vi "Panel Split Engine.vi"() -> ()   [LabVIEW 2016]
uses:
  PanelRootNode.lvclass
  QueueManager.llb/Destroy.vi
  QueueManager.llb/Remove.vi
  PanelDataNode/PanelDataNode.lvclass
  QueueManager.llb/CreatQueue.vi
  <vilib>/Utility/error.llb/DialogType.ctl
panel:
  out "RootNode*":refnum<data-value>
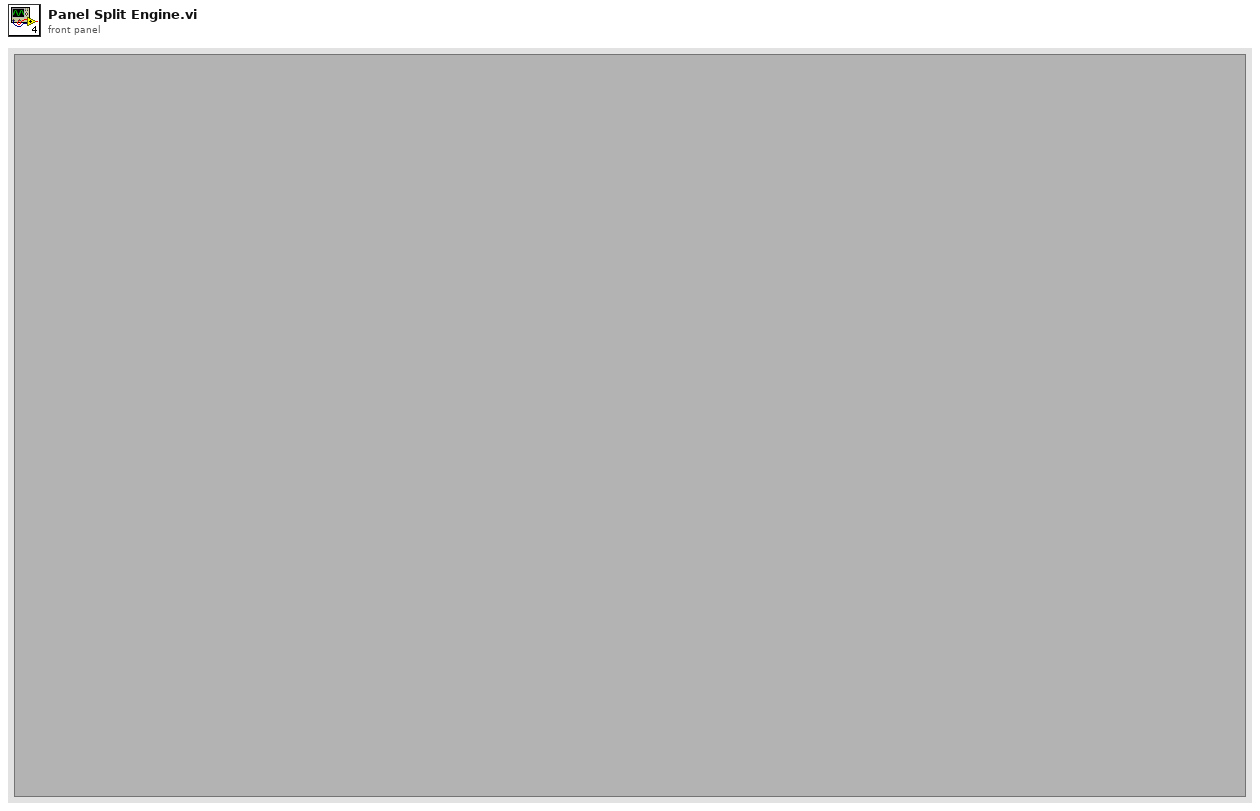
[diagram p1: front panel]
types:
  T1 = cluster{"error":errorcluster, "Event":string, "Data":variant, "Q_Local":string, "RootNode*":refnum<data-value>, "Caller":string}
  T2 = typedef "DialogType.ctl" = u16
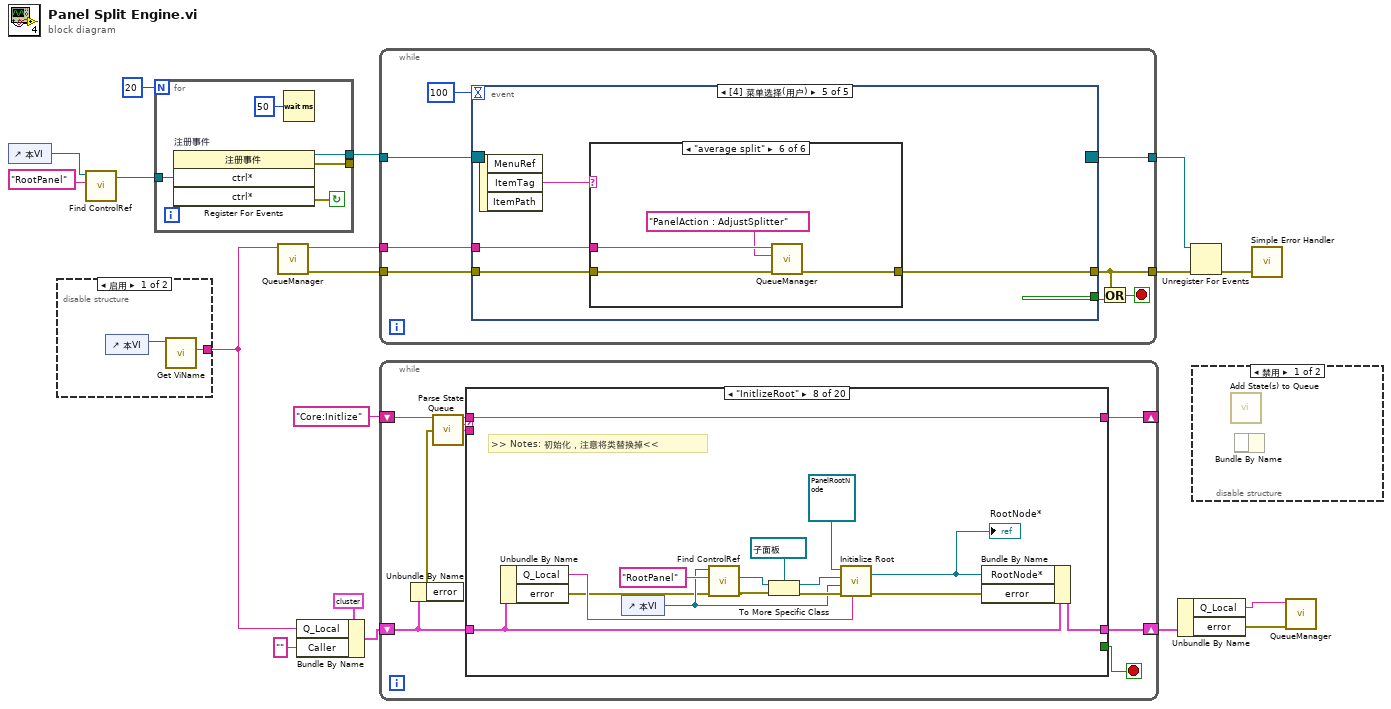
[diagram p0: block diagram]
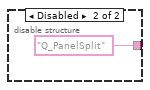
[diagram p2: hidden frame]
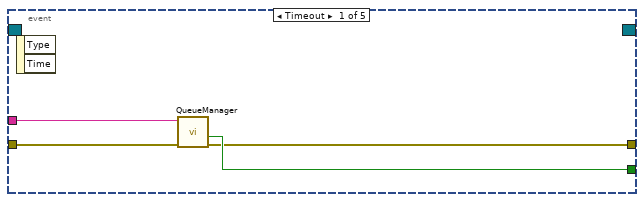
[diagram p4: hidden frame]
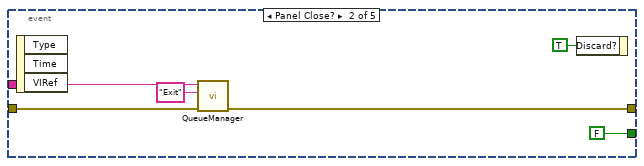
[diagram p5: hidden frame]
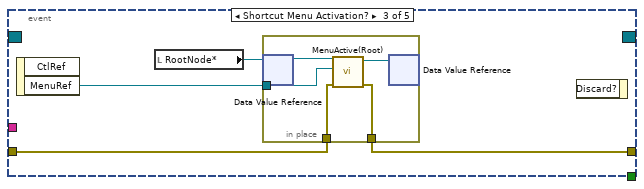
[diagram p6: hidden frame]
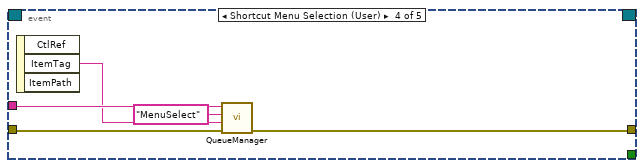
[diagram p7: hidden frame]
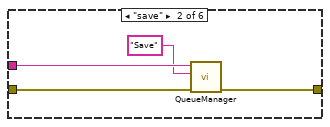
[diagram p9: hidden frame]
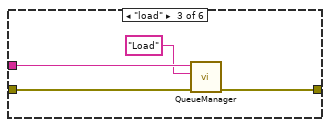
[diagram p10: hidden frame]
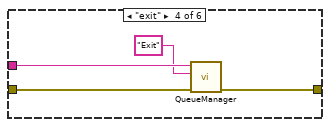
[diagram p11: hidden frame]
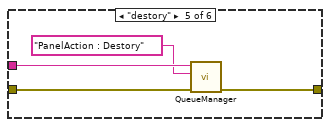
[diagram p12: hidden frame]
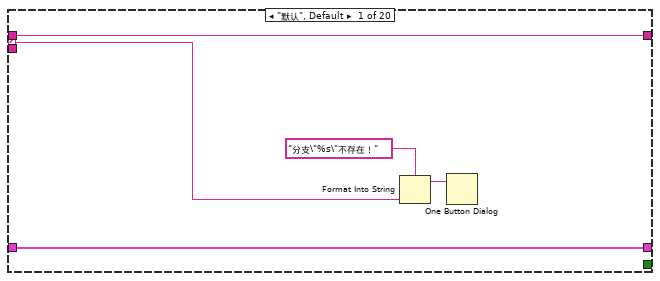
[diagram p13: hidden frame]
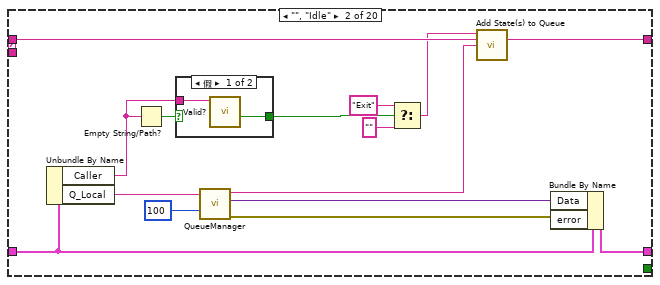
[diagram p14: hidden frame]
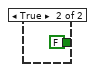
[diagram p15: hidden frame]
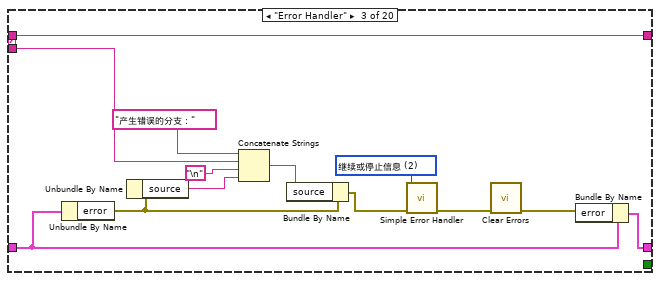
[diagram p16: hidden frame]
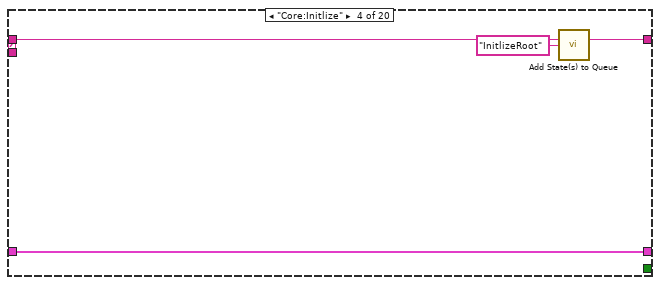
[diagram p17: hidden frame]
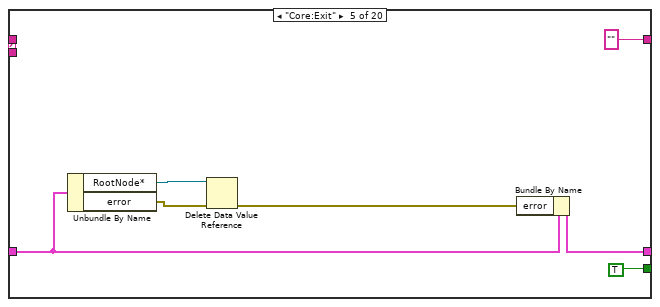
[diagram p18: hidden frame]
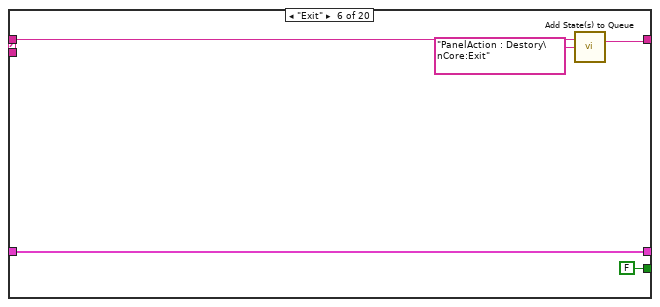
[diagram p19: hidden frame]
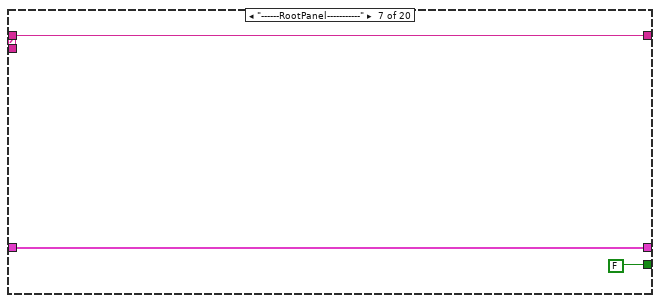
[diagram p20: hidden frame]
diagram:
  n1 = control-ref of="本VI"() -> (w8:refnum<vi>)
  n2 = disable-structure shown="启用" {
    disable-tunnel: [w18 "Q_PanelSplit" ("QueueName")] -> w10
    frame Enabled {
      n3 = control-ref of="本VI"() -> (w19:refnum<vi>)
      n4 = call "Get ViName.vi"("VI*"=w19) -> ("VI Name"=w18:string)  [unwired: 8 in, 2 out]
    }
    frame Disabled {
    }
  }
  n5 = call "Find ControlRef.vi"("control name"="RootPanel", "vi*"=w8) -> ("ctrl*"=w2:refnum<vi>)  [unwired: 7 in, 2 out]
  n6 = for {
    N: 20 -> [_]
    tunnel: [w22] -> _
    tunnel: [w24] -> w3
    tunnel: w2 -> [w23]
    stop <- w22 continue-if-true
    n7 = register-events "注册事件"(w23, w23) -> (reference out=w24:refnum<event-registration>, error out=w22:errorcluster)  [unwired: 2 in]
    n8 = Wait (ms)(milliseconds to wait=u32 50 ("等待时间（毫秒）")) -> ()  [unwired: 1 out]
  }
  n9 = call-poly "QueueManager.vi"("QueueName"=w10) -> ("error out"=w17:errorcluster)  [unwired: 9 in, 1 out]
  n10 = Bundle By Name(cluster=T1 {"error"={"status"=FALSE, "code"=0, "source"=""}, "Event"="", "Data"=variant, "Q_Local"="", "RootNode*"=refnum, "Caller"=""} ("TmpData"), "Q_Local"=w10, "Caller"="") -> (w12:T1)
  n11 = while {
    tunnel: w17 -> [w31]
    tunnel: w10 -> [w32]
    tunnel: [w28] -> w6
    tunnel: w3 -> [w26]
    tunnel: [w25] -> w4
    stop <- w29 stop-if-true
    n12 = event shown="[4] 菜单选择(用户)" {
      selector: w26 -> [_ _ _ _ _]
      dyn-events: [_ _ _ _ _] -> w25
      timeout: 100 -> [_ _ _ _ _]
      tunnel: [w34 FALSE _ _ _] -> w30
      tunnel: w32 -> [w36 w41 _ w56 w59]
      tunnel: w31 -> [w35 w40 w45 w55 w58]
      tunnel: [w33 w39 w46 w54 w57] -> w28
      event Timeout {
        n13 = event-data() -> ()  [unwired: 1 in, 2 out]
        n14 = call-poly "QueueManager.vi"("error in (no error)"=w35, "Queue Name(unamed)"=w36) -> ("error out"=w33:errorcluster, "Not Exist?"=w34:bool)  [unwired: 8 in]
      }
      event Panel Close? {
        n15 = event-data() -> ()  [unwired: 1 in, 3 out]
        n16 = call-poly "QueueManager.vi"("error in"=w40, "Event"="Exit", "QueueName"=w41) -> ("error out"=w39:errorcluster)  [unwired: 7 in, 1 out]
        n17 = event-data("Discard?"=TRUE ("放弃？")) -> ()  [unwired: 1 in, 1 out]
      }
      event Shortcut Menu Activation? {
        n18 = event-data() -> ("MenuRef"=w44:refnum<k9>)  [unwired: 1 in, 1 out]
        n19 = local read "RootNode*"() -> (w43:refnum<data-value>)
        n20 = in-place {
          in-place-border: w44 -> [w49]
          in-place-border: w45 -> [w48]
          in-place-border: [w47] -> w46
          n21 = in-place-dvr #1(w43) -> (w51:refnum<class "PanelRootNode.lvclass">)  [unwired: 1 out]
          n22 = call "MenuActive(Root).vi"("error in (no error)"=w48, "菜单引用"=w49, "PanelDataNode 输入"=w51) -> ("error out"=w47:errorcluster, "PanelDataNode 输出"=w50:refnum<class "PanelRootNode.lvclass">)  [unwired: 7 in]
          n23 = in-place-dvr #1(w50) -> ()  [unwired: 2 out]
        }
        n24 = event-data() -> ()  [unwired: 2 in, 1 out]
      }
      event Shortcut Menu Selection (User) {
        n25 = event-data() -> ("ItemTag"=w53:string)  [unwired: 1 in, 2 out]
        n26 = call-poly "QueueManager.vi"("error in"=w55, "Data"=w53, "Event"="MenuSelect", "QueueName"=w56) -> ("error out"=w54:errorcluster)  [unwired: 6 in, 1 out]
      }
      event Menu Selection (User) {
        n27 = event-data() -> ("ItemTag"=w60:string)  [unwired: 1 in, 2 out]
        n28 = case shown="\"average split\"" w60 {
          tunnel: w59 -> [_ w65 w69 w73 w77 w81]
          tunnel: w58 -> [w61 w63 w67 w71 w75 w79]
          tunnel: [w61 w62 w66 w70 w74 w78] -> w57
          frame "假", Default {
          }
          frame "save" {
            n29 = call-poly "QueueManager.vi"("error in"=w63, "Event"="Save", "QueueName"=w65) -> ("error out"=w62:errorcluster)  [unwired: 7 in, 1 out]
          }
          frame "load" {
            n30 = call-poly "QueueManager.vi"("error in"=w67, "Event"="Load", "QueueName"=w69) -> ("error out"=w66:errorcluster)  [unwired: 7 in, 1 out]
          }
          frame "exit" {
            n31 = call-poly "QueueManager.vi"("error in"=w71, "Event"="Exit", "QueueName"=w73) -> ("error out"=w70:errorcluster)  [unwired: 7 in, 1 out]
          }
          frame "destory" {
            n32 = call-poly "QueueManager.vi"("error in"=w75, "Event"="PanelAction : Destory", "QueueName"=w77) -> ("error out"=w74:errorcluster)  [unwired: 7 in, 1 out]
          }
          frame "average split" {
            n33 = call-poly "QueueManager.vi"("error in"=w79, "Event"="PanelAction : AdjustSplitter", "QueueName"=w81) -> ("error out"=w78:errorcluster)  [unwired: 7 in, 1 out]
          }
        }
      }
    }
    n34 = Or(x=w28, y=w30) -> (x .or. y?=w29:bool)
  }
  n35 = while {
    shift-right: [w83] -> w14
    shift-left: w12 -> [w84]
    shift-right: [w82] -> _
    shift-left: "Core:Initlize" -> [w90]
    stop <- w86 stop-if-true
    n36 = Unbundle By Name(w84) -> ("error"=w85:errorcluster)
    n37 = call "Parse State Queue.vi"("State Queue"=w90, "Error In (no error)"=w85) -> ("Remaining States"=w89:string, "Current State"=w88:string, "Arguments"=w87:string)  [unwired: 10 in, 1 out]
    n38 = case shown="\"InitlizeRoot\"" w88 {
      selector: w88 -> [w91 _ _ _ _ _ _ _ _ _ _ _ _ _ _ _ _ _ _ _]
      tunnel: w89 -> [w94 w106 w126 w129 _ w142 w143 w160 w168 w189 w207 w219 w230 w237 w248 w258 w268 w278 w284 w296]
      tunnel: w87 -> [_ _ w114 _ _ _ _ _ _ _ _ _ _ _ _ _ _ _ _ _]
      tunnel: [_ _ _ _ TRUE FALSE FALSE _ _ _ _ _ _ _ _ _ _ _ _ _] -> w86
      tunnel: w84 -> [w95 w103 w116 w130 w133 w139 w144 w152 w170 w187 w205 w223 w229 w236 w246 w256 w266 w276 w283 w294]
      tunnel: [w95 w109 w115 w130 w132 w139 w144 w154 w169 w186 w204 w222 w229 w235 w245 w255 w265 w275 w283 w293] -> w83
      tunnel: [w94 w105 w126 w128 "" ("Remaining States") w141 w143 w160 w168 w189 w207 w218 w230 w237 w248 w258 w268 w278 w284 w296] -> w82
      frame "默认", Default {
        n39 = Format Into String(format string="分支\"%s\"不存在！" ("格式字符串"), w91) -> (resulting string=w93:string)  [unwired: 2 in, 1 out]
        n40 = One Button Dialog(message=w93) -> ()  [unwired: 1 in, 1 out]
      }
      frame "", "Idle" {
        n41 = Unbundle By Name(w103) -> ("Caller"=w97:string, "Q_Local"=w102:string)
        n42 = Empty String/Path?(string/path=w97) -> (empty?=w101:bool)
        n43 = case shown="假" w101 {
          tunnel: [w112 FALSE ("Not Exist?")] -> w100
          tunnel: w97 -> [w111 _]
          frame False {
            n44 = call "Valid?.vi"("Queue Name(unamed)"=w111) -> ("Not Exist?"=w112:bool)  [unwired: 9 in, 1 out]
          }
          frame True {
          }
        }
        n45 = call-poly "QueueManager.vi"("Time out(-1)"=100, "Queue Name"=w102) -> ("error out"=w110:errorcluster, "Data"=w108:variant, "Event"=w107:string)  [unwired: 6 in, 1 out]
        n46 = Select(t="Exit" ("Event"), s=w100, f="") -> (s? t:f=w96:string)
        n47 = call "Add State(s) to Queue.vi"("State(s) in Front (\"\")"=w96, "State(s) in (\"\")"=w106, "State(s) at Back (\"\")"=w107) -> ("States Out"=w105:string)  [unwired: 12 in]
        n48 = Bundle By Name(cluster=w103, "Data"=w108, "error"=w110) -> (w109:T1)
      }
      frame "Error Handler" {
        w123 = T2 2 items=["无对话框", "确定信息", "继续或停止信息", "确定信息＋警告", "继续/停止+警告"] ("type of dialog (OK msg:1)")
        n49 = Unbundle By Name(w116) -> ("error"=w118:errorcluster)
        n50 = Unbundle By Name(w118) -> ("source"=w121:string)
        n51 = Concatenate Strings("产生错误的分支：" ("字符串"), w114, "\n", w121) -> (w119:string)
        n52 = Bundle By Name(cluster=w118, "source"=w119) -> (w117:errorcluster)
        n53 = call <vilib>:"Simple Error Handler.vi"("type of dialog (OK msg:1)"=w123, "error in (no error)"=w117) -> ("error out"=w124:errorcluster)  [unwired: 3 in, 4 out]
        n54 = call <vilib>:"Clear Errors.vi"("error in (no error)"=w124) -> ("error out"=w125:errorcluster)  [unwired: 5 in, 1 out]
        n55 = Bundle By Name(cluster=w116, "error"=w125) -> (w115:T1)
      }
      frame "Core:Initlize" {
        n56 = call "Add State(s) to Queue.vi"("State(s) in (\"\")"=w129, "State(s) at Back (\"\")"="InitlizeRoot" ("State(s) at Back (\"\")")) -> ("States Out"=w128:string)  [unwired: 13 in]
      }
      frame "Core:Exit" {
        n57 = Unbundle By Name(w133) -> ("RootNode*"=w135:refnum<data-value>, "error"=w131:errorcluster)
        n58 = Delete Data Value Reference(data value reference=w135, error in=w131) -> (error out=w134:errorcluster)  [unwired: 1 out]
        n59 = Bundle By Name(cluster=w133, "error"=w134) -> (w132:T1)
      }
      frame "Exit" {
        n60 = call "Add State(s) to Queue.vi"("State(s) in (\"\")"=w142, "State(s) at Back (\"\")"="PanelAction : Destory\nCore:Exit" ("State(s) at Back (\"\")")) -> ("States Out"=w141:string)  [unwired: 13 in]
      }
      frame "------RootPanel-----------" {
      }
      frame "InitlizeRoot" {
        # ">> Notes: 初始化，注意将类替换掉<<"
        n61 = Unbundle By Name(w152) -> ("Q_Local"=w151:string, "error"=w146:errorcluster)
        n62 = control-ref of="本VI"() -> (w147:refnum<vi>)
        n63 = call "Find ControlRef.vi"("error in (no error)"=w146, "control name"="RootPanel", "vi*"=w147) -> ("error out"=w149:errorcluster, "ctrl*"=w148:refnum<vi>)  [unwired: 6 in, 1 out]
        n64 = To More Specific Class(target class=refnum<vi> refnum ("RootPanel"), reference=w148, error in=w149) -> (specific class reference=w157:refnum<vi>, error out=w156:errorcluster)
        n65 = call-dynamic "Initialize Root.vi"("RootQueueName"=w151, "error in (no error)"=w156, "CurrentVi*"=w147, "RootPanel*"=w157, "PanelRootNode 输入"=refnum<class "PanelRootNode.lvclass"> refnum ("PanelRootNode.lvclass")) -> ("error out"=w155:errorcluster, "SelfNode*"=w153:refnum<data-value>)  [unwired: 5 in]
        "RootNode*" <- w153
        n66 = Bundle By Name(cluster=w152, "RootNode*"=w153, "error"=w155) -> (w154:T1)
      }
      frame "Save" {
        # ">> Notes: 保存分割结果，可通过队列发送保存的路径，也可不发送路径，自动弹出文件选择对话框。<<"
        n67 = Unbundle By Name(w170) -> ("RootNode*"=w171:refnum<data-value>, "Data"=w166:variant, "error"=w161:errorcluster)
        n68 = Variant To Data(error in=w161, type=path "" ("路径"), Variant=w166) -> (data=w164:path, error out=w163:errorcluster)
        n69 = call <vilib>:"Clear Errors.vi"("error in (no error)"=w163) -> ("error out"=w162:errorcluster)  [unwired: 5 in, 1 out]
        n70 = in-place {
          in-place-border: [w174] -> w167
          in-place-border: w164 -> [w173]
          in-place-border: w162 -> [w172]
          n71 = in-place-dvr #2(w171) -> (w176:refnum<class "PanelRootNode.lvclass">)  [unwired: 1 out]
          n72 = call-dynamic "Save Xml.vi"("error in"=w172, "selected path"=w173, "PanelRootNode 输入"=w176) -> ("error out"=w174:errorcluster, "PanelRootNode 输出"=w175:refnum<class "PanelRootNode.lvclass">)  [unwired: 7 in]
          n73 = in-place-dvr #2(w175) -> ()  [unwired: 2 out]
        }
        n74 = Bundle By Name(cluster=w170, "error"=w167) -> (w169:T1)
      }
      frame "Load" {
        n75 = Unbundle By Name(w187) -> ("RootNode*"=w188:refnum<data-value>, "Data"=w183:variant, "error"=w180:errorcluster)
        n76 = Variant To Data(error in=w180, type=path "" ("路径"), Variant=w183) -> (data=w182:path, error out=w184:errorcluster)
        n77 = call <vilib>:"Clear Errors.vi"("error in (no error)"=w184) -> ("error out"=w181:errorcluster)  [unwired: 5 in, 1 out]
        n78 = in-place {
          in-place-border: [w193] -> w178
          in-place-border: w182 -> [w191]
          in-place-border: w181 -> [w190]
          n79 = in-place-dvr #3(w188) -> (w192:refnum<class "PanelRootNode.lvclass">)  [unwired: 1 out]
          n80 = call-dynamic "Load Xml.vi"("error in"=w190, "selected path"=w191, "PanelRootNode 输入"=w192) -> ("error out"=w193:errorcluster, "PanelRootNode 输出"=w194:refnum<class "PanelRootNode.lvclass">)  [unwired: 7 in]
          n81 = in-place-dvr #3(w194) -> (w179:errorcluster)  [unwired: 1 out]
        }
        n82 = Merge Errors(w179, w178) -> (w177:errorcluster)
        n83 = Bundle By Name(cluster=w187, "error"=w177) -> (w186:T1)
      }
      frame "LoadXmlString" {
        n84 = Unbundle By Name(w205) -> ("RootNode*"=w206:refnum<data-value>, "Q_Local"=w195:string, "Data"=w202:variant, "error"=w199:errorcluster)
        n85 = Variant To Data(error in=w199, type=w195, Variant=w202) -> (data=w201:string, error out=w203:errorcluster)
        n86 = call <vilib>:"Clear Errors.vi"("error in (no error)"=w203) -> ("error out"=w200:errorcluster)  [unwired: 5 in, 1 out]
        n87 = in-place {
          in-place-border: [w211] -> w197
          in-place-border: w201 -> [w208]
          in-place-border: w200 -> [w212]
          n88 = in-place-dvr #4(w206) -> (w210:refnum<class "PanelRootNode.lvclass">)  [unwired: 1 out]
          n89 = call-dynamic "LoadXmlString.vi"("error in"=w212, "XmlString"=w208, "PanelRootNode 输入"=w210) -> ("error out"=w211:errorcluster, "PanelRootNode 输出"=w209:refnum<class "PanelRootNode.lvclass">)  [unwired: 7 in]
          n90 = in-place-dvr #4(w209) -> (w198:errorcluster)  [unwired: 1 out]
        }
        n91 = Merge Errors(w198, w197) -> (w196:errorcluster)
        n92 = Bundle By Name(cluster=w205, "error"=w196) -> (w204:T1)
      }
      frame "MenuSelect" {
        n93 = Unbundle By Name(w223) -> ("RootNode*"=w217:refnum<data-value>, "Data"=w221:variant, "error"=w213:errorcluster)
        n94 = Variant To Data(error in=w213, type="", Variant=w221) -> (data=w216:string, error out=w215:errorcluster)
        n95 = in-place {
          in-place-border: w216 -> [w226]
          in-place-border: w215 -> [w225]
          in-place-border: [w224] -> w214
          n96 = in-place-dvr #5(w217) -> (w228:refnum<class "PanelRootNode.lvclass">)  [unwired: 1 out]
          n97 = call-dynamic "MenuSelect.vi"("error in"=w225, "Tag"=w226, "PanelRootNode 输入"=w228) -> ("error out"=w224:errorcluster, "PanelRootNode 输出"=w227:refnum<class "PanelRootNode.lvclass">)  [unwired: 7 in]
          n98 = in-place-dvr #5(w227) -> ()  [unwired: 2 out]
        }
        n99 = Bundle By Name(cluster=w223, "error"=w214) -> (w222:T1)
        n100 = call "Add State(s) to Queue.vi"("State(s) in (\"\")"=w219) -> ("States Out"=w218:string)  [unwired: 14 in]
      }
      frame "-------PanelAction----------" {
      }
      frame "PanelAction : Split" {
        n101 = Unbundle By Name(w236) -> ("RootNode*"=w234:refnum<data-value>, "Data"=w233:variant, "error"=w231:errorcluster)
        n102 = in-place {
          in-place-border: w233 -> [w240]
          in-place-border: [w239] -> w232
          in-place-border: w231 -> [w238]
          n103 = in-place-dvr #6(w234) -> (w242:refnum<class "PanelRootNode.lvclass">)  [unwired: 1 out]
          n104 = call-dynamic "Split.vi"("error in"=w238, "Data"=w240, "PanelRootNode 输入"=w242) -> ("error out"=w239:errorcluster, "PanelRootNode 输出"=w241:refnum<class "PanelRootNode.lvclass">)  [unwired: 7 in]
          n105 = in-place-dvr #6(w241) -> ()  [unwired: 2 out]
        }
        n106 = Bundle By Name(cluster=w236, "error"=w232) -> (w235:T1)
      }
      frame "PanelAction : Delete" {
        n107 = Unbundle By Name(w246) -> ("RootNode*"=w247:refnum<data-value>, "Data"=w244:variant)
        n108 = in-place {
          in-place-border: w244 -> [w250]
          in-place-border: [w249] -> w243
          n109 = in-place-dvr #7(w247) -> (w252:refnum<class "PanelRootNode.lvclass">)  [unwired: 1 out]
          n110 = call-dynamic "Delete.vi"("Data"=w250, "PanelRootNode 输入"=w252) -> ("error out"=w249:errorcluster, "PanelRootNode 输出"=w251:refnum<class "PanelRootNode.lvclass">)  [unwired: 8 in]
          n111 = in-place-dvr #7(w251) -> ()  [unwired: 2 out]
        }
        n112 = Bundle By Name(cluster=w246, "error"=w243) -> (w245:T1)
      }
      frame "PanelAction : Insert" {
        n113 = Unbundle By Name(w256) -> ("RootNode*"=w257:refnum<data-value>, "Data"=w253:variant)
        n114 = in-place {
          in-place-border: [w259] -> w254
          in-place-border: w253 -> [w260]
          n115 = in-place-dvr #8(w257) -> (w262:refnum<class "PanelRootNode.lvclass">)  [unwired: 1 out]
          n116 = call-dynamic "Insert.vi"("Data"=w260, "PanelRootNode 输入"=w262) -> ("error out"=w259:errorcluster, "PanelRootNode 输出"=w261:refnum<class "PanelRootNode.lvclass">)  [unwired: 8 in]
          n117 = in-place-dvr #8(w261) -> ()  [unwired: 2 out]
        }
        n118 = Bundle By Name(cluster=w256, "error"=w254) -> (w255:T1)
      }
      frame "PanelAction : Destory" {
        # ">> Notes: 销毁分割结果，回到最初状态<<"
        n119 = Unbundle By Name(w266) -> ("RootNode*"=w267:refnum<data-value>, "error"=w263:errorcluster)
        n120 = in-place {
          in-place-border: [w270] -> w264
          in-place-border: w263 -> [w269]
          n121 = in-place-dvr #9(w267) -> (w272:refnum<class "PanelRootNode.lvclass">)  [unwired: 1 out]
          n122 = call-dynamic "Destory.vi"("error in (no error)"=w269, "PanelRootNode 输入"=w272) -> ("error out"=w270:errorcluster, "PanelRootNode 输出"=w271:refnum<class "PanelRootNode.lvclass">)  [unwired: 8 in]
          n123 = in-place-dvr #9(w271) -> ()  [unwired: 2 out]
        }
        n124 = Bundle By Name(cluster=w266, "error"=w264) -> (w265:T1)
      }
      frame "PanelAction : AdjustSplitter" {
        # ">> Notes: 均分面板<<"
        n125 = Unbundle By Name(w276) -> ("RootNode*"=w277:refnum<data-value>, "error"=w273:errorcluster)
        n126 = in-place {
          in-place-border: [w280] -> w274
          in-place-border: w273 -> [w279]
          n127 = in-place-dvr #10(w277) -> (w282:refnum<class "PanelRootNode.lvclass">)  [unwired: 1 out]
          n128 = call "Adjust Splitter.vi"("error in (no error)"=w279, "PanelRootNode 输入"=w282) -> ("error out"=w280:errorcluster, "PanelRootNode 输出"=w281:refnum<class "PanelRootNode.lvclass">)  [unwired: 8 in]
          n129 = in-place-dvr #10(w281) -> ()  [unwired: 2 out]
        }
        n130 = Bundle By Name(cluster=w276, "error"=w274) -> (w275:T1)
      }
      frame "------Communication---------" {
      }
      frame "SendToAll" {
        # ">> Notes: 发送至所有面板中插入的VI线程，要求插入的VI使用的队列名是VI名称；<<"
        n131 = Unbundle By Name(w294) -> ("RootNode*"=w295:refnum<data-value>, "Data"=w291:variant, "error"=w285:errorcluster)
        n132 = Variant To Data(error in=w285, type=cluster{"Event":string, "Data":variant} {"Event"="", "Data"=variant}, Variant=w291) -> (data=w289:cluster{"Event":string, "Data":variant}, error out=w286:errorcluster)
        n133 = Unbundle By Name(w289) -> ("Event"=w288:string, "Data"=w287:variant)
        n134 = in-place {
          in-place-border: [w301] -> w292
          in-place-border: w288 -> [w300]
          in-place-border: w287 -> [w299]
          in-place-border: w286 -> [w298]
          n135 = in-place-dvr #11(w295) -> (w303:refnum<class "PanelRootNode.lvclass">)  [unwired: 1 out]
          n136 = call "SendToPanels.vi"("PanelNumber(-1)"=-1, "error in"=w298, "Data"=w299, "Event"=w300, "PanelRootNode in"=w303) -> ("error out"=w301:errorcluster, "PanelRootNode out"=w302:refnum<class "PanelRootNode.lvclass">)  [unwired: 5 in]
          n137 = in-place-dvr #11(w302) -> ()  [unwired: 2 out]
        }
        n138 = Bundle By Name(cluster=w294, "error"=w292) -> (w293:T1)
      }
    }
  }
  n139 = Unbundle By Name(w14) -> ("Q_Local"=w11:string, "error"=w15:errorcluster)
  n140 = Unregister For Events(event registration refnum=w4, error in=w6) -> (error out=w5:errorcluster)
  n141 = disable-structure shown="禁用" {
    frame Disabled {
      n142 = call "Add State(s) to Queue.vi"() -> ()  [unwired: 15 in, 1 out]
      n143 = Bundle By Name() -> ()  [unwired: 2 in, 1 out]
    }
    frame Enabled {
    }
  }
  n144 = call <vilib>:"Simple Error Handler.vi"("error in (no error)"=w5) -> ()  [unwired: 4 in, 5 out]
  n145 = call-poly "QueueManager.vi"("error in (no error)"=w15, "QueeuName"=w11) -> ()  [unwired: 9 in, 1 out]
